vi "ReadFifo.vi"(8 "error in (no error)":errorcluster, 10 "N":i32, 11 "FPGA_Concrete in":refnum<class "FPGA_Concrete.lvclass">) -> (0 "error out":errorcluster, 2 "Data":dbl[](array[numeric]), 3 "FPGA_Concrete out":refnum<class "FPGA_Concrete.lvclass">)   [LabVIEW 2019, in "FPGA_Concrete.lvclass"]
uses:
  FPGA_Concrete.lvclass
  FPGA_Concrete.lvclass/FPGA_Concrete.ctl
  <vilib>/Utility/error.llb/Error Cluster From Error Code.vi
  <vilib>/rvi/errors/niLvFpgaAdjustHostInterfaceError.vi
  <vilib>/rvi/interface/nirviMethod/nirviMethod.xnode
  FPGA VI Reference.ctl
  <vilib>/FPGAPlugInAG/Dynamic/niLvFpga_ReadFifo_Dynamic.vi
  <vilib>/rvi/errors/niLvFpgaMergeErrorWithErrorCode.vi
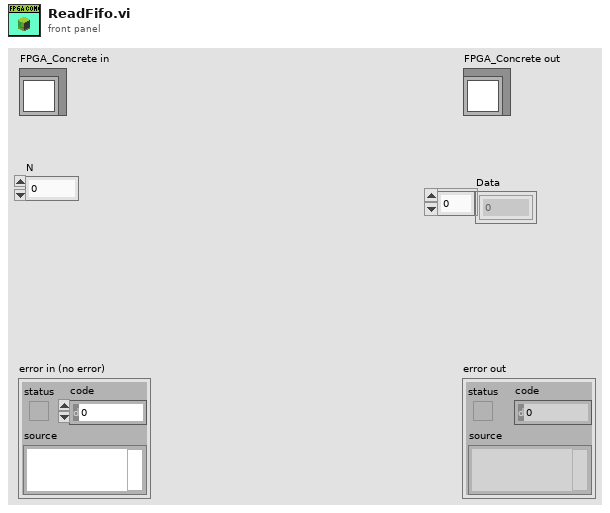
[diagram p1: front panel]
types:
  T1 = typedef "FPGA_Concrete.lvclass/FPGA VI Reference.ctl" = refnum<k20>
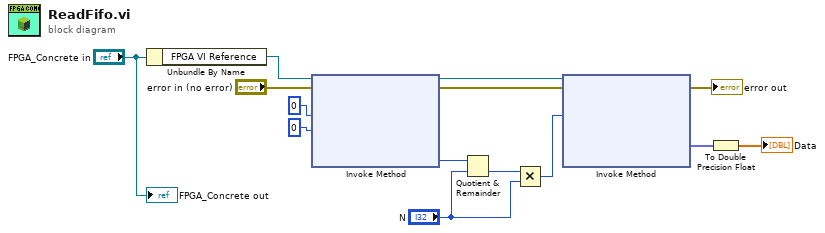
[diagram p0: block diagram]
diagram:
  n1 = Unbundle By Name("FPGA_Concrete in") -> ("FPGA VI Reference"=w13:T1)
  n2 = xnode "Invoke Method"("FPGA VI Reference In"=w13, "error in"="error in (no error)", "Number of Elements"=u32 0, "Timeout (ms)"=0) -> ("FPGA VI Reference Out"=w6:T1, "error out"=w5:errorcluster, "Elements Remaining"=w9:u32)  [unwired: 1 out]
  n3 = Quotient & Remainder(x=w9, y="N") -> (floor(x/y)=w10:u32)  [unwired: 1 out]
  n4 = Multiply(x=w10, y="N") -> (x*y=w7:u32)
  n5 = xnode "Invoke Method"("FPGA VI Reference In"=w6, "error in"=w5, "Number of Elements"=w7) -> ("error out"=→"error out":errorcluster, "Data"=w2:fxp<+/-,21,-4>[])  [unwired: 1 in, 2 out]
  n6 = To Double Precision Float(number=w2) -> (double precision float=→"Data":dbl[])
  "FPGA_Concrete out" <- "FPGA_Concrete in"
